vi "Read coeffs.vi"(8 "error in (no error)":errorcluster, 11 "Polynomial Scale configuration in":refnum<class "Polynomial Scale configuration.lvclass">) -> (0 "error out":errorcluster, 2 "coeff sets":cluster{"coeffs":dbl[]}[](array[cluster]), 3 "Polynomial Scale configuration out":refnum<class "Polynomial Scale configuration.lvclass">)   [LabVIEW 2013, in "Polynomial Scale configuration.lvclass"]
uses:
  Polynomial Scale configuration.lvclass
  Polynomial Scale configuration.lvclass/Polynomial Scale configuration.ctl
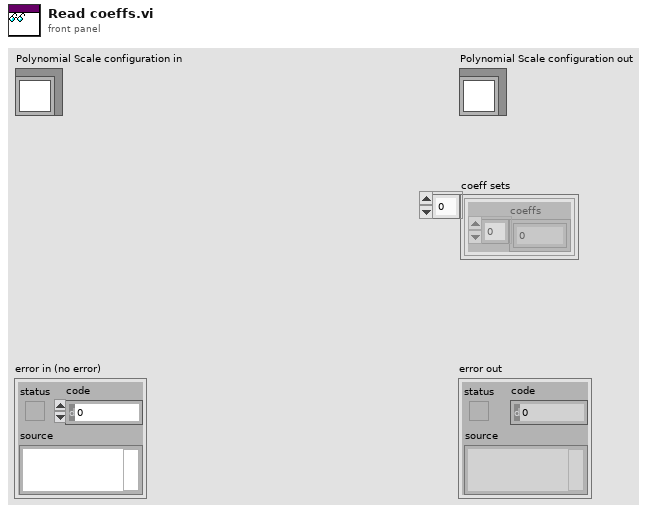
[diagram p1: front panel]
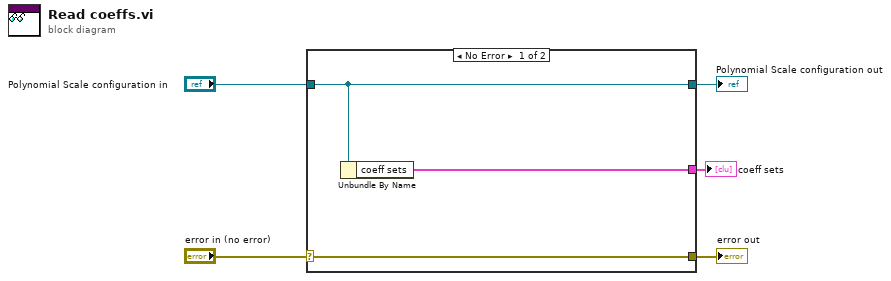
[diagram p0: block diagram]
diagram:
  n1 = case shown="No Error" "error in (no error)" {
    selector: "error in (no error)" -> [w8 w9]
    tunnel: [w8 w9] -> w4
    tunnel: [w7 w10] -> w2
    tunnel: "Polynomial Scale configuration in" -> [w7 w10]
    tunnel: [w6 _] -> w1
    frame No Error {
      n2 = Unbundle By Name(w7) -> ("coeff sets"=w6:cluster{"coeffs":dbl[]}[])
    }
    frame Error {
    }
  }
  "error out" <- w4
  "Polynomial Scale configuration out" <- w2
  "coeff sets" <- w1
